vi "Get Code.vi"(8 "error in (no error)":errorcluster, 11 "UIMessage in":refnum<class "UIMessage.lvclass">) -> (0 "error out":errorcluster, 2 "Code":T1, 3 "UIMessage out":refnum<class "UIMessage.lvclass">)   [LabVIEW 2020, in "TSnax.lvlib" / "UIMessage.lvclass"]
uses:
  UIMessage.lvclass
  UIMessage.lvclass/UIMessage.ctl
  UIMsg.ctl
  TSnax.lvlib
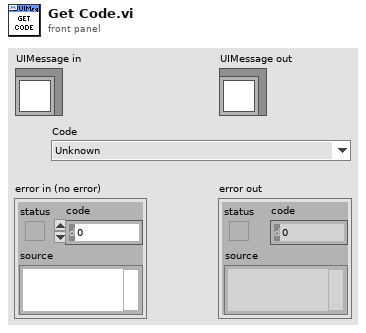
[diagram p1: front panel]
types:
  T1 = typedef "TSnax.lvlib/UIMsg.ctl" = enum16{"Unknown", "BreakOnUserRequest", "BreakOnBreakpoint", "BreakOnRunTimeError", "Trace", "TerminatingExecution", "AbortingExecution", "KillingExecutionThreads", "EndExecution", "ShutDownComplete", "StartExecution", "ProgressPercent", "ProgressText", "StartInteractiveExecution", "EndInteractiveExecution", "TerminatingInteractiveExecution", "TerminationCancelled", "ResumeFromBreak", "StartFileExecution", "EndFileExecution", "ShutDownCancelled", "LocalizationSettingChanged", "OpenWindows", "TileWindows", "CascadeWindows", "ReportChanged", "CloseWindows", "RefreshWindows", "ClientFileChanged", "DisplayReport", "ModelState_Initializing", "ModelState_Waiting", "ModelState_Identified", "ModelState_BeginTesting", "ModelState_TestingComplete", "ModelState_PostProcessingComplete", "ModelState_EnabledStateSet", "ReportLocationChanged", "GotoLocation", "PushUndoItem", "OutputMessages", "TypePaletteFileListChanged", "NonTerminatingThreadsArePreventingTermination", "ModelState_PostProcessing", "ReportCollectionChanged", "RuntimeError"}
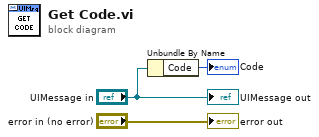
[diagram p0: block diagram]
diagram:
  n1 = Unbundle By Name("UIMessage in") -> ("Code"=→"Code":T1)
  "error out" <- "error in (no error)"
  "UIMessage out" <- "UIMessage in"
